vi "Run Configuration Script.vi"(0 "fpga interface in":refnum<k20>, 5 "serial channels":string[](array[string]), 7 "configuration script":path, 11 "error in (no error)":errorcluster) -> (4 "fpga interface out":refnum<k20>, 15 "error out":errorcluster)   [LabVIEW 2025]
uses:
  <instrlib>/FlexRIO/Automotive Vision Utility/v1/Host/Automotive Vision Utility.lvlib
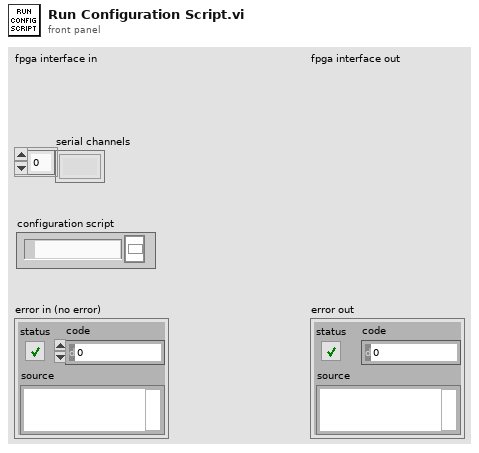
[diagram p1: front panel]
types:
  T1 = typedef "Automotive Vision Utility.lvlib/SerDes Configuration Command.ctl" = cluster{"command type":T2, "address":u16, "write data":u8[], "num bytes to read":u32, "milliseconds to wait":u32}
  T2 = typedef "Automotive Vision Utility.lvlib/SerDes Configuration Command Type.ctl" = enum16{"Wait", "Write", "Transfer", "Read"}
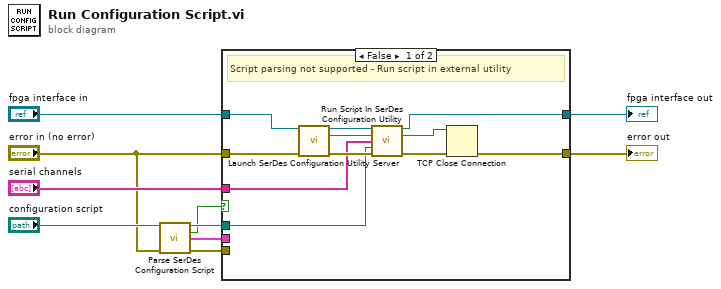
[diagram p0: block diagram]
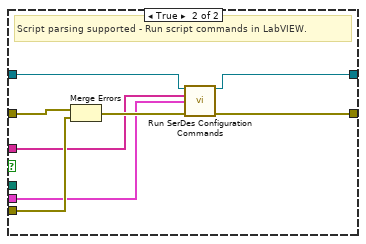
[diagram p2: hidden frame]
diagram:
  n1 = call <instrlib>:"Parse SerDes Configuration Script.vi"("configuration script"="configuration script", "error in"="error in (no error)") -> ("configuration script out"=w5:path, "file type supported?"=w1:bool, "serdes config commands"=w4:T1[], "error out"=w3:errorcluster)  [unwired: 10 in]
  n2 = case shown="False" w1 {
    tunnel: "fpga interface in" -> [w21 w24]
    tunnel: "error in (no error)" -> [w20 w28]
    tunnel: "serial channels" -> [w16 w22]
    tunnel: w5 -> [w15 _]
    tunnel: [w12 w29] -> w8
    tunnel: [w11 w23] -> w7
    tunnel: w4 -> [_ w25]
    tunnel: w3 -> [_ w26]
    frame False {
      # "Script parsing not supported - Run script in external utility"
      n3 = call <instrlib>:"Launch SerDes Configuration Utility Server.vi"("fpga interface in"=w21, "error in"=w20) -> ("fpga interface out"=w19:refnum<k20>, "socket connection id out"=w18:refnum<k5>, "error out"=w17:errorcluster)  [unwired: 11 in]
      n4 = call <instrlib>:"Run Script In SerDes Configuration Utility.vi"("fpga interface in"=w19, "socket connection id in"=w18, "serial channels"=w16, "configuration script"=w15, "error in"=w17) -> ("fpga interface out"=w11:refnum<k20>, "socket connection id out"=w14:refnum<k5>, "error out"=w13:errorcluster)  [unwired: 8 in]
      n5 = TCP Close Connection(connection ID=w14, error in (no error)=w13) -> (error out=w12:errorcluster)  [unwired: 1 in, 1 out]
    }
    frame True {
      # "Script parsing supported - Run script commands in LabVIEW."
      n6 = Merge Errors(w28, w26) -> (w27:errorcluster)
      n7 = call <instrlib>:"Run SerDes Configuration Commands.vi"("fpga interface in"=w24, "serial channels"=w22, "serdes config commands"=w25, "error in"=w27) -> ("fpga interface out"=w23:refnum<k20>, "error out"=w29:errorcluster)  [unwired: 9 in, 1 out]
    }
  }
  "fpga interface out" <- w7
  "error out" <- w8
